vi "SearchConfigurationSectionName.vi"(10 "Secetion Array":string[][](array[string])=[["Boolean_Data", "BD1", "BD2", "BD3", "BD4"], ["Double_Data", "DD1", "DD2", "DD3", "DD4"], ["I32_Data", "ID1", "ID2", "ID3", "ID4"], ["Path_Data", "PD1", "PD2", "", ""], ["String_Data", "SD1", "SD2", "", ""], ["U32_Data", "UD1", "UD2", "UD3", "UD4"]], 11 "KeyName":string="PD2") -> (3 "Section":string)   [LabVIEW 2015]
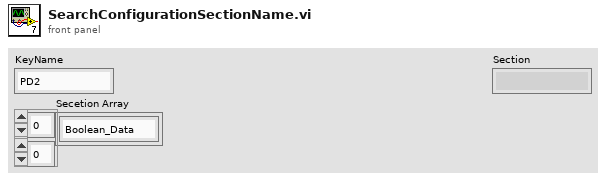
[diagram p1: front panel]
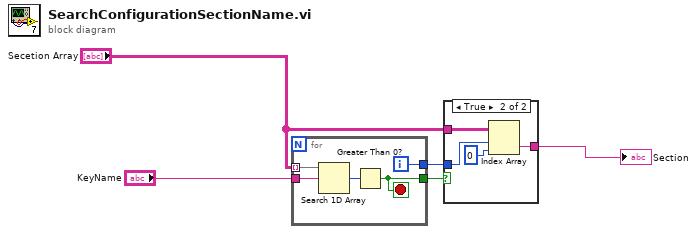
[diagram p0: block diagram]
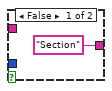
[diagram p2: hidden frame]
diagram:
  n1 = for {
    tunnel: "Secetion Array" -> [w10] mode=indexing
    tunnel: "KeyName" -> [w9]
    tunnel: [w7] -> w3
    tunnel: [w6] -> w2
    i -> [w7]
    stop <- w6 stop-if-true
    n2 = Search 1D Array(1D array=w10, element=w9) -> (index of element=w8:i32)  [unwired: 1 in]
    n3 = Greater Than 0?(x=w8) -> (x > 0?=w6:bool)
  }
  n4 = case shown="True" w2 {
    tunnel: "Secetion Array" -> [_ w15]
    tunnel: w3 -> [_ w14]
    tunnel: ["Section" ("String") w12] -> w1
    frame False {
    }
    frame True {
      n5 = Index Array(array=w15, index (row)=w14, index (col)=0 ("disabled index (col)")) -> (element=w12:string)
    }
  }
  "Section" <- w1
